vi "ASI_init.vi"(2 "error in (no error)":errorcluster, 3 "timeout (ms)":u32=100, 4 "VISA resource name":refnum<visa-resource-name>="COM7") -> (0 "error out":errorcluster, 1 "VISA resource name out":refnum<visa-resource-name>)   [LabVIEW 2015]
doc: "Establishes connection with configured port (default = COM1).\nSends command MOVE X=x Y=y where x and y are integers denoting 10ths of a micron.\nSub-VI SerialWaitForStatusN.vi polls controller with STATUS command until 'N' (not busy) status is returned, or until a configured maximum number of unsuccessful tries (default = 400).\nDisconnects from configured port."
uses:
  <vilib>/Instr/_visa.llb/VISA Configure Serial Port (Instr).vi
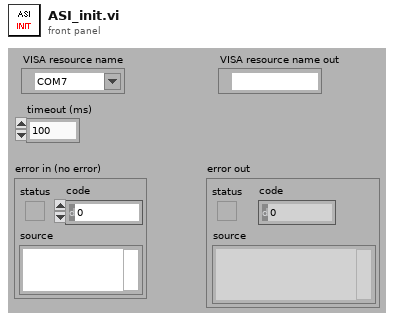
[diagram p1: front panel]
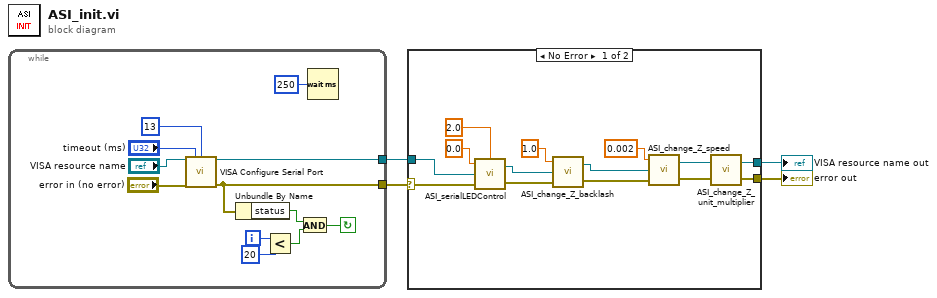
[diagram p0: block diagram]
diagram:
  n1 = while {
    tunnel: [w11] -> w1
    tunnel: [w12] -> w4
    i -> [w10]
    stop <- w6 continue-if-true
    n2 = call-poly "VISA Configure Serial Port"("VISA resource name"="VISA resource name", "timeout (10sec)"="timeout (ms)", "termination char\n(0xA = '\\n' = LF)"=u8 13 ("termination char\n(0xA = '\\n' = LF)"), "error in (no error)"="error in (no error)") -> ("VISA resource name out"=w12:refnum<visa-resource-name>, "error out"=w11:errorcluster)  [unwired: 10 in]
    n3 = Unbundle By Name(w11) -> ("status"=w8:bool)
    n4 = Less?(x=w10, y=20) -> (x < y?=w7:bool)
    n5 = And(x=w8, y=w7) -> (x .and. y?=w6:bool)
    n6 = Wait (ms)(milliseconds to wait=u32 250) -> ()  [unwired: 1 out]
  }
  n7 = case shown="No Error" w1 {
    selector: w1 -> [w18 w31]
    tunnel: w4 -> [w24 w32]
    tunnel: [w20 w31] -> w3
    tunnel: [w19 w32] -> w2
    frame No Error {
      n8 = call "ASI_serialLEDControl.vi"("Delay Time (s)"=2.0, "error in (no error)"=w18, "VISA resource name"=w24, "setpoint"=0.0) -> ("error out"=w29:errorcluster, "VISA resource name out"=w23:refnum<visa-resource-name>)
      n9 = call "ASI_change_Z_backlash.vi"("error in (no error)"=w29, "VISA resource name"=w23, "backlash (um)"=1.0) -> ("error out"=w26:errorcluster, "VISA resource name out"=w22:refnum<visa-resource-name>)
      n10 = call "ASI_change_Z_speed.vi"("error in (no error)"=w26, "VISA resource name"=w22, "speed"=0.002) -> ("error out"=w25:errorcluster, "VISA resource name out"=w21:refnum<visa-resource-name>)
      n11 = call "ASI_change_Z_unit_multiplier.vi"("error in (no error)"=w25, "VISA resource name"=w21) -> ("error out"=w20:errorcluster, "VISA resource name out"=w19:refnum<visa-resource-name>)
    }
    frame Error {
    }
  }
  "VISA resource name out" <- w2
  "error out" <- w3
